vi "dvp Vi Set Ae Operation.vi"(10 "AeOperation":u32(ring) items=["AE_OP_OFF", "AE_OP_ONCE", "AE_OP_CONTINUOUS"], 11 "handle":u32) -> (3 "function return":u32(ring))   [LabVIEW 2018, in "LabViewDVPCamera.lvlib"]
doc: "LabviewDvp2Api dvpStatus dvpViSetAeOperation(dvpHandle handle, dvpAeOperation AeOperation);"
uses:
  LabViewDVPCamera.lvlib
  LabViewDVPCamera/LabViewDVPCamera.dll
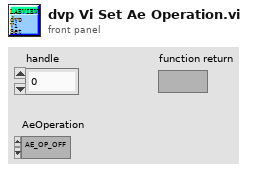
[diagram p1: front panel]
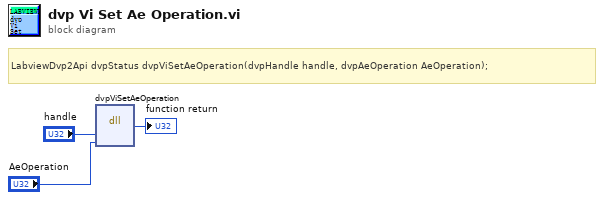
[diagram p0: block diagram]
diagram:
  # "LabviewDvp2Api dvpStatus dvpViSetAeOperation(dvpHandle handle, dvpAeOperation AeOperation);"
  n1 = dll-call lib="C:/Program Files (x86)/DVP2 Labview cn 64/Sample/LabViewDVPCamera/LabViewDVPCamera.*" fn="dvpViSetAeOperation"("handle"="handle", "AeOperation"="AeOperation") -> (→"function return":u32)  [unwired: 5 in, 2 out]
